vi "N Array Resigter.vi"(8 "error in (no error)":errorcluster, 10 "Event Source":string[](array[string]), 11 "Taget":string) -> (0 "error out":errorcluster)   [LabVIEW 2020]
uses:
  <userlib>/_NEVSTOP/Communicable State Machine(CSM)/_Polymophic/CSM - Replace Mark with String Array.vi
  <userlib>/_NEVSTOP/Communicable State Machine(CSM)/Communicable State Machine.lvlib
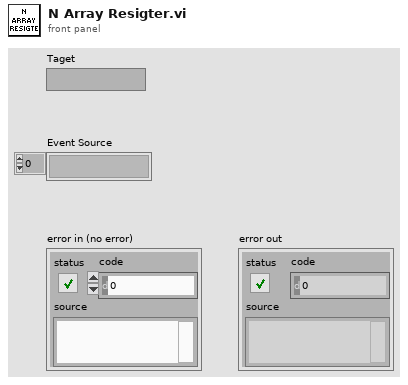
[diagram p1: front panel]
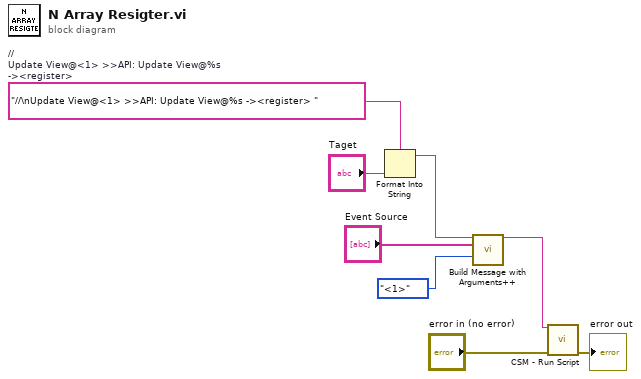
[diagram p0: block diagram]
diagram:
  w5 = "//\nUpdate View@<1> >>API: Update View@%s -><register> "  # // Update View@<1> >>API: Update View@%s -><register>
  n1 = Format Into String(format string=w5, "Taget") -> (resulting string=w4:string)  [unwired: 2 in, 1 out]
  n2 = call-poly <userlib>:"Build Message with Arguments++.vi"("Single-line Text"=w4, "Replace String"="Event Source", "Substitution Mark"=enum16{"<1>", "<2>", "<3>", "<4>"}."<1>") -> ("States"=w1:string)  [unwired: 12 in]
  n3 = call <userlib>:"CSM - Run Script.vi"("CSM Scripts"=w1, "error in (no error)"="error in (no error)") -> ("error out"=→"error out":errorcluster)  [unwired: 11 in, 2 out]
